vi "Get Limit State.vi"(8 "error in (no error)":errorcluster, 10 "Limit Line (1: Line1)":u16(ring)=1 items=["Line1"=1, "Line2"=2], 11 "VISA resource name":refnum<visa-resource-name>) -> (0 "error out":errorcluster, 2 "Pass?":bool, 3 "VISA resource name out":refnum<visa-resource-name>)   [LabVIEW 2014, in "Agilent ESA PSA Series.lvlib"]
doc: "Queries the status of limit line testing."
uses:
  Agilent ESA PSA Series.lvlib
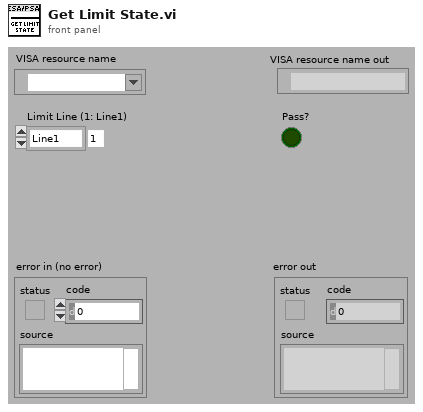
[diagram p1: front panel]
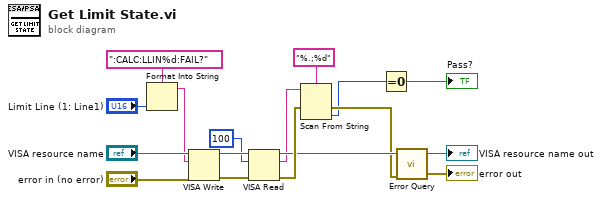
[diagram p0: block diagram]
diagram:
  n1 = Format Into String(format string=":CALC:LLIN%d:FAIL?", "Limit Line (1: Line1)") -> (resulting string=w14:string)  [unwired: 2 in, 1 out]
  n2 = VISA Write(VISA resource name="VISA resource name", write buffer=w14, error in (no error)="error in (no error)") -> (VISA resource name out=w13:refnum<visa-resource-name>, error out=w12:errorcluster)  [unwired: 1 out]
  n3 = VISA Read(VISA resource name=w13, byte count=u32 100, error in (no error)=w12) -> (VISA resource name out=w6:refnum<visa-resource-name>, read buffer=w4:string, error out=w10:errorcluster)  [unwired: 1 out]
  n4 = Scan From String(format string="%.;%d", input string=w4, error in=w10) -> (error out=w5:errorcluster, output 1=w3:i32)  [unwired: 2 in, 2 out]
  n5 = Equal To 0?(x=w3) -> (x = 0?=→"Pass?":bool)
  n6 = call "Error Query.vi"("error in (no error)"=w5, "VISA resource name"=w6) -> ("error out"=→"error out":errorcluster, "VISA resource name out"=→"VISA resource name out":refnum<visa-resource-name>)  [unwired: 6 in, 2 out]
